vi "Boolean cluster to number.vi"(11 "Output Channel Enable":T1) -> (3 "Numeric":u32)   [LabVIEW 2012]
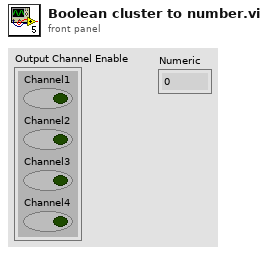
[diagram p1: front panel]
types:
  T1 = cluster{"Channel1":bool, "Channel2":bool, "Channel3":bool, "Channel4":bool}
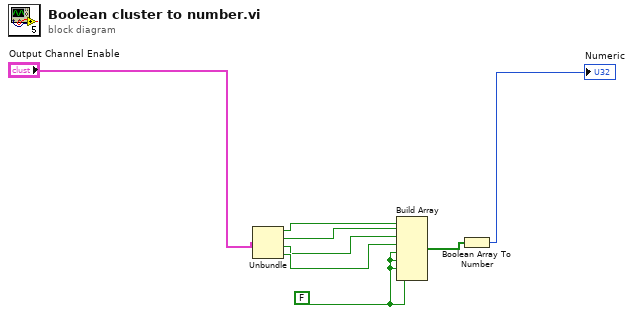
[diagram p0: block diagram]
diagram:
  w1 = FALSE ("element")
  n1 = Unbundle("Output Channel Enable") -> ("Channel1"=w4:bool, "Channel2"=w5:bool, "Channel3"=w6:bool, "Channel4"=w7:bool)
  n2 = Build Array(w4, w5, w6, w7, w1, w1, w1, w1) -> (w2:bool[])
  n3 = Boolean Array To Number(Boolean array=w2) -> (number=→"Numeric":u32)
